vi "NIVS PWM In.vi"(2 "PWM In Timeout":u32, 3 "FPGA I/O":refnum<k21>) -> (0 "PWM In Freq Packet":u64, 1 "PWM In DC Packet":u64)   [LabVIEW 2010]
uses:
  <vilib>/eio/EIONode/EIONode.xnode
  <vilib>/rvi/eio/nirviEIOImplementation/nirviEIOImplementation.xnode
  <vilib>/rvi/eio/common/nirviEmuClasses.ctl
  <vilib>/rvi/eio/common/nirviEmuTemplateMethod_noerrors.vi
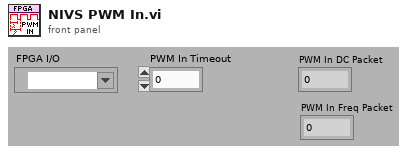
[diagram p1: front panel]
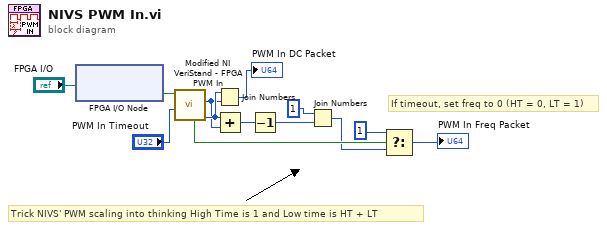
[diagram p0: block diagram]
diagram:
  # "If timeout, set freq to 0 (HT = 0, LT = 1)"
  # "Trick NIVS' PWM scaling into thinking High Time is 1 and Low time is HT + LT"
  n1 = xnode "FPGA I/O Node"("FPGA I/O In"="FPGA I/O") -> ("I/O Item"=w10:bool)  [unwired: 1 out]
  n2 = call "Modified NI VeriStand - FPGA PWM In.vi"("Time Out"="PWM In Timeout", "Value"=w10) -> ("High time"=w12:u32, "Low Time"=w11:u32, "Timeout?"=w5:bool)  [unwired: 7 out]
  n3 = Join Numbers(hi=w12, lo=w11) -> ((hi.lo)=→"PWM In DC Packet":u64)
  n4 = Add(x=w12, y=w11) -> (x+y=w7:u32)
  n5 = Decrement(x=w7) -> (x-1=w6:u32)
  n6 = Join Numbers(hi=u32 1, lo=w6) -> ((hi.lo)=w3:u64)
  n7 = Select(t=u64 1 ("(hi.lo)"), s=w5, f=w3) -> (s? t:f=→"PWM In Freq Packet":u64)
